vi "WriteReadWait.vi"(5 "Read Value":bool=TRUE, 7 "Write Value":bool=TRUE, 8 "error in (no error)":errorcluster, 9 "Read":i32, 10 "Write":i32, 11 "I-O in":refnum<class "I-O.lvclass">) -> (0 "error out":errorcluster, 3 "I-O out":refnum<class "I-O.lvclass">)   [LabVIEW 2018, in "I-O.lvclass"]
uses:
  I-O.lvclass
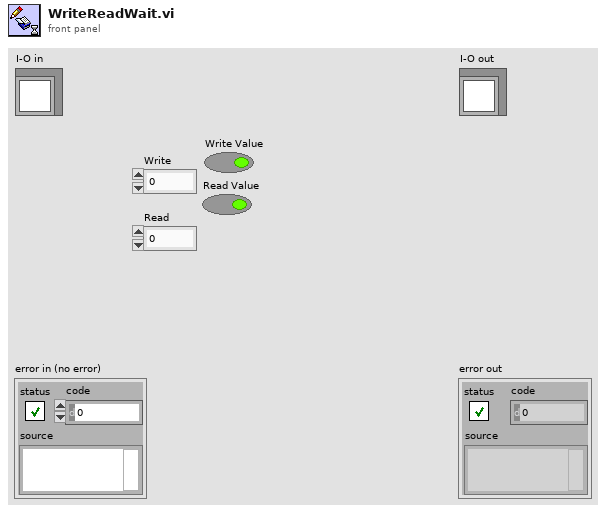
[diagram p1: front panel]
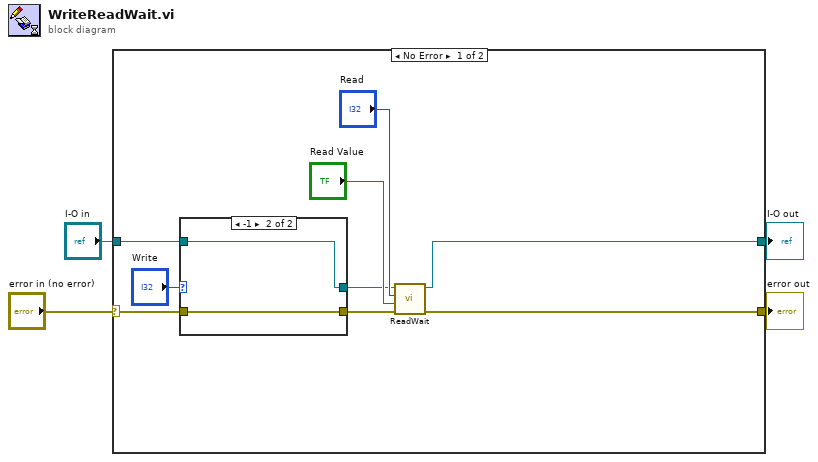
[diagram p0: block diagram]
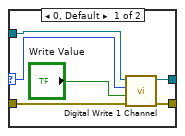
[diagram p2: hidden frame]
diagram:
  n1 = case shown="No Error" "error in (no error)" {
    selector: "error in (no error)" -> [w10 w23]
    tunnel: [w11 w23] -> w3
    tunnel: [w12 w22] -> w1
    tunnel: "I-O in" -> [w13 w22]
    frame No Error {
      n2 = case shown="-1" "Write" {
        selector: "Write" -> [w14 _]
        tunnel: w13 -> [w19 w20]
        tunnel: w10 -> [w18 w21]
        tunnel: [w16 w20] -> w7
        tunnel: [w15 w21] -> w6
        frame 0, Default {
          n3 = call-dynamic "Digital Write 1 Channel.vi"("error constant"=w18, "Value"="Write Value", "Channel"=w14, "I-O.lvclass"=w19) -> ("error IO"=w15:errorcluster, "I-O.lvclass 2"=w16:refnum<class "I-O.lvclass">)  [unwired: 6 in]
        }
        frame -1 {
        }
      }
      n4 = call "ReadWait.vi"("error in (no error)"=w6, "Value"="Read Value", "Read"="Read", "I-O in"=w7) -> ("error out"=w11:errorcluster, "I-O out"=w12:refnum<class "I-O.lvclass">)  [unwired: 6 in]
    }
    frame Error {
    }
  }
  "error out" <- w3
  "I-O out" <- w1
